vi "Write Comms Event.vi"(8 "error in (no error)":errorcluster, 10 "Comms Event":refnum<user-event>, 11 "LED Matrix in":refnum<class "LED Matrix.lvclass">) -> (0 "error out":errorcluster, 3 "LED Matrix out":refnum<class "LED Matrix.lvclass">)   [LabVIEW 2026, in "LED Matrix.lvlib" / "LED Matrix.lvclass"]
uses:
  LED Matrix.lvclass
  LED Matrix.lvclass/LED Matrix.ctl
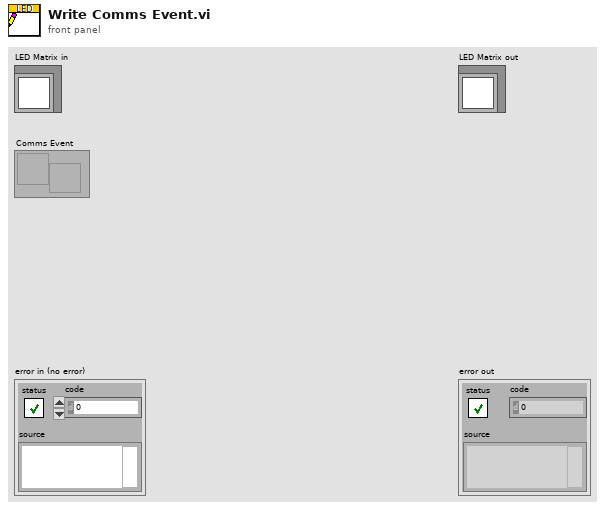
[diagram p1: front panel]
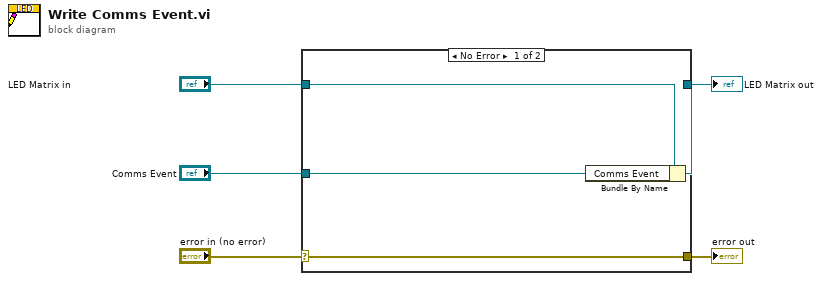
[diagram p0: block diagram]
diagram:
  n1 = case shown="No Error" "error in (no error)" {
    selector: "error in (no error)" -> [w9 w10]
    tunnel: [w9 w10] -> w4
    tunnel: [w7 w11] -> w2
    tunnel: "LED Matrix in" -> [w8 w11]
    tunnel: "Comms Event" -> [w6 _]
    frame No Error {
      n2 = Bundle By Name(cluster=w8, "Comms Event"=w6) -> (w7:refnum<class "LED Matrix.lvclass">)
    }
    frame Error {
    }
  }
  "error out" <- w4
  "LED Matrix out" <- w2
